vi "Yaw Zero.vi"(11 "Angle":dbl) -> ()   [LabVIEW 2015]
uses:
  Robot Global Data.vi
  navX.Library.v2/navX Library v2/navX Library v2.lvlib
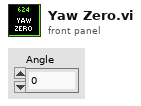
[diagram p1: front panel]
types:
  T1 = typedef "navX Library v2.lvlib/Z900_navX_DeviceTypeDef.ctl" = cluster{"Interface":cluster{"Protocol":T2, "Update Rate (4Hz-60Hz)":u8, "navX Open TypeDef":variant}, "Notify Packet":refnum<notifier>, "Loop VI Refnum":refnum<vi>, "Ready to Close Occurrence Refnum":refnum<k4>}
  T2 = typedef "navX Library v2.lvlib/Z900_navX_ProtocolTypeDef.ctl" = enum16{"SERIAL", "I2C", "SPI"}
  T3 = cluster{"Yaw":dbl, "Roll":dbl, "Pitch":dbl, "Heading":dbl, "Fused Heading":dbl}
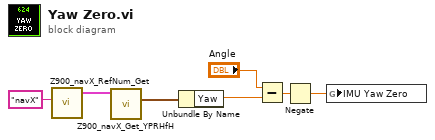
[diagram p0: block diagram]
diagram:
  n1 = call "Z900_navX_RefNum_Get.vi"("refnum name"="navX") -> ("navX Device"=w1:T1)  [unwired: 9 in, 1 out]
  n2 = call "Z900_navX_Get_YPRHfH.vi"("navX Device"=w1) -> ("YRPHfH"=w6:T3)  [unwired: 7 in, 3 out]
  n3 = Unbundle By Name(w6) -> ("Yaw"=w5:dbl)
  n4 = Subtract(x="Angle", y=w5) -> (x-y=w3:dbl)
  n5 = Negate(x=w3) -> (-x=w2:dbl)
  n6 = global write "Robot Global Data.vi" "IMU Yaw Zero"(w2) -> ()
